vi "Read Mapping.vi"(8 "error in (no error)":errorcluster, 11 "MLTFNC in":refnum<class "MLTFNC.lvclass">) -> (0 "error out":errorcluster, 2 "Mapping":T1, 3 "MLTFNC out":refnum<class "MLTFNC.lvclass">)   [LabVIEW 2019, in "MLTFNC.lvlib" / "MLTFNC.lvclass"]
uses:
  Library/MLTFNC.lvclass
  Custom Controls/Mapping.ctl
  Library/MLTFNC.lvclass/MLTFNC.ctl
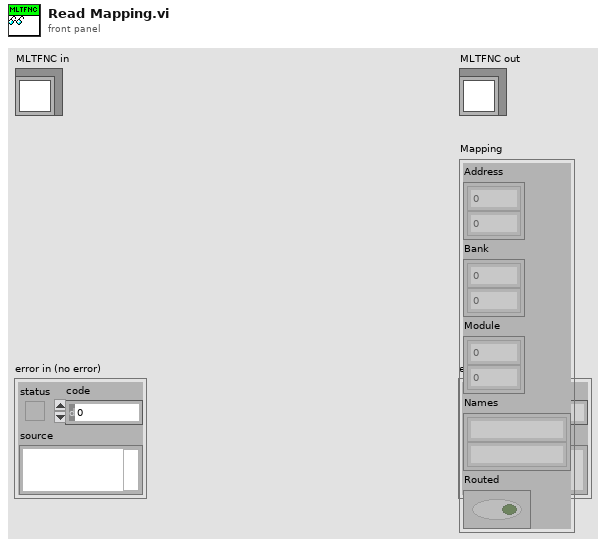
[diagram p1: front panel]
types:
  T1 = typedef "MLTFNC.lvlib/MLTFNC.lvclass/Mapping.ctl" = cluster{"Address":u32[], "Bank":u32[], "Module":u32[], "Names":string[], "Routed":bool[]}
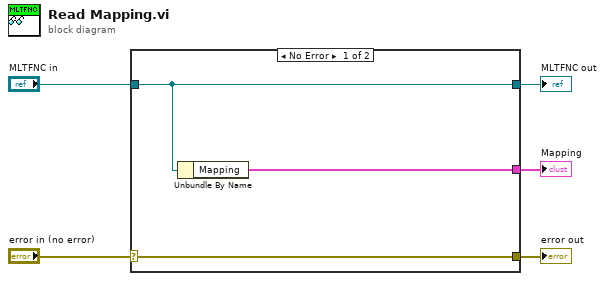
[diagram p0: block diagram]
diagram:
  n1 = case shown="No Error" "error in (no error)" {
    selector: "error in (no error)" -> [w8 w9]
    tunnel: [w8 w9] -> w4
    tunnel: [w7 w10] -> w2
    tunnel: "MLTFNC in" -> [w7 w10]
    tunnel: [w6 _] -> w1
    frame No Error {
      n2 = Unbundle By Name(w7) -> ("Mapping"=w6:T1)
    }
    frame Error {
    }
  }
  "error out" <- w4
  "MLTFNC out" <- w2
  "Mapping" <- w1
